vi "Int Saving.vi"(11 "Cluster":T1) -> (1 "Data.txt":path, 2 "created path":path, 3 "Byte Stream File out":refnum<file>)   [LabVIEW 2018]
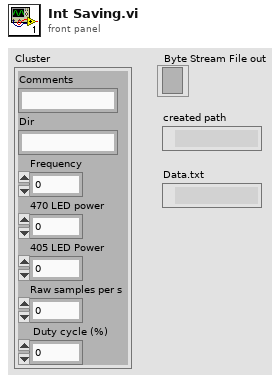
[diagram p1: front panel]
types:
  T1 = cluster{"Comments":string, "Dir":string, "Frequency":dbl, "470 LED power":dbl, "405 LED Power":dbl, "Raw samples per s":dbl, " Duty cycle (%)":dbl}
  T2 = enum16{"open", "replace", "create", "open or create", "replace or create", "replace or create with confirmation"}
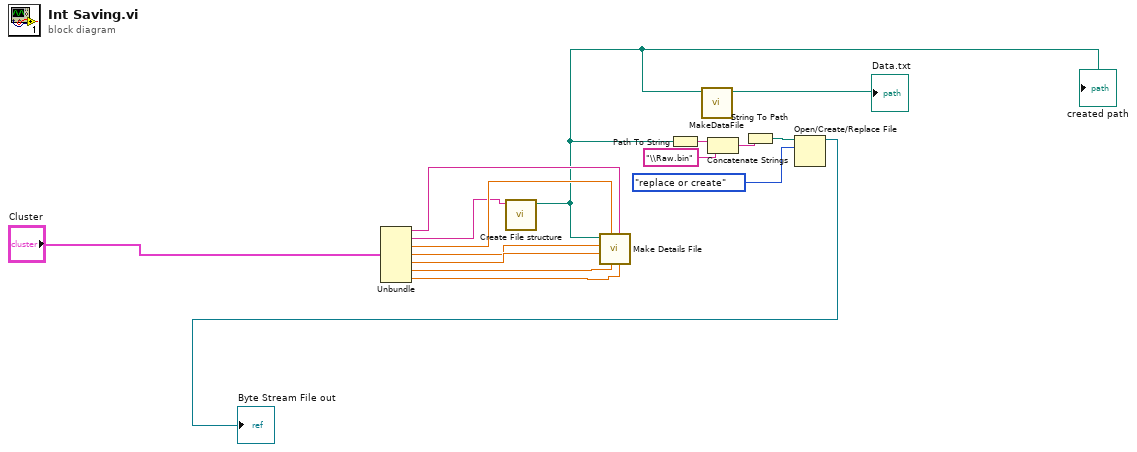
[diagram p0: block diagram]
diagram:
  n1 = Unbundle("Cluster") -> ("Comments"=w11:string, "Dir"=w10:string, "Frequency"=w12:dbl, "470 LED power"=w13:dbl, "405 LED Power"=w14:dbl, "Raw samples per s"=w15:dbl, "Duty cycle (%)"=w16:dbl)
  n2 = call "Create File structure.vi"("Dir"=w10) -> ("created path"=w8:path)  [unwired: 10 in]
  "created path" <- w8
  n3 = call "Make Details File.vi"("Duty cycle (%)"=w16, "Comments"=w11, "Number of samples per s"=w15, "Frequency"=w12, "405 LED Power"=w14, "470 LED power"=w13, "created path"=w8) -> ()  [unwired: 5 in]
  n4 = Path To String(path=w8) -> (string=w2:string)
  n5 = call "MakeDataFile.vi"("created path"=w8) -> ("Path"=→"Data.txt":path)  [unwired: 10 in]
  n6 = Concatenate Strings(w2, "\\Raw.bin" ("string")) -> (w3:string)
  n7 = String To Path(string=w3) -> (path=w5:path)
  n8 = Open/Create/Replace File(file path (use dialog)=w5, operation (0:open)=T2."replace or create") -> (refnum out=→"Byte Stream File out":refnum<file>)  [unwired: 4 in, 2 out]
